vi "rad_GetImageFolderRoot.vi"(4 "error in":errorcluster, 7 "Image Path":path) -> (0 "error out":errorcluster, 1 "directory":bool, 2 "ImageFolderRoot":path, 3 "Image Path out":path)   [LabVIEW 2023]
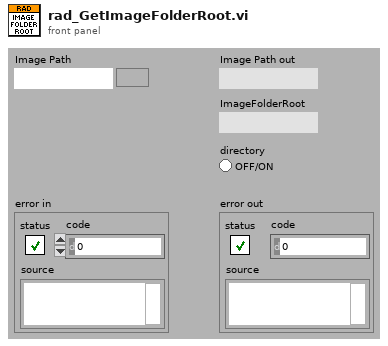
[diagram p1: front panel]
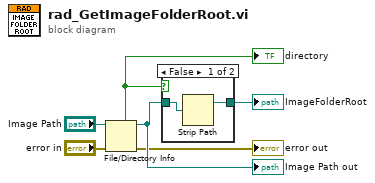
[diagram p0: block diagram]
diagram:
  n1 = File/Directory Info(path="Image Path", error in="error in") -> (path out=w6:path, directory=w1:bool, error out=→"error out":errorcluster)  [unwired: 4 out]
  "Image Path out" <- w6
  "directory" <- w1
  n2 = case shown="False" w1 {
    tunnel: w6 -> [w8 w9]
    tunnel: [w7 w9] -> w5
    frame False {
      n3 = Strip Path(path=w8) -> (stripped path=w7:path)  [unwired: 1 out]
    }
    frame True {
    }
  }
  "ImageFolderRoot" <- w5
